vi "Periodic Tasks.vi"(8 "error in (no error)":errorcluster) -> ()   [LabVIEW 2023]
doc: "This VI runs in parallel to other tasks. It can contain as many user-defined periodic loops as you need. These can carry out PID or other sorts of timed response."
uses:
  Drive/DriveGlobal.vi
  <vilib>/Rock Robotics/Network Tables/NT Read String.vi
  <vilib>/Rock Robotics/Network Tables/NT Write Number.vi
  <vilib>/Rock Robotics/Network Tables/NT Write String.vi
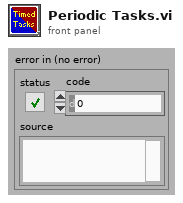
[diagram p1: front panel]
types:
  T1 = typedef "ADIS16470 Device Reference.ctl" = cluster{"DevStatus":errorcluster, "Hardware Config":T2, "Calibration Complete":refnum<notifier>, "Status Reference":refnum<data-value>, "Data Reference":refnum<data-value>, "Sychronous Process VI":T6, "Cmd FIFO":refnum<k33>, "Source":T7, "Data FIFO":refnum<k33>, "Calibration Time (ms)":u32, "Data Reference":refnum<data-value>}
  T2 = typedef "ADIS16470 Hardware Configuration.ctl" = cluster{"SPI Clock Rate (Hz)":dbl, "IMU SPI Mode (3)":T3, "IMU Reset Pin":T4, "IMU SPI Bus":T5, "IMU Data Ready Pin":T4, "Stall Config":cluster{"Pow2BytesPerRead":u8, "StallTicks":u16, "CsToSclkTicks":u8}}
  T3 = typedef "WPI_SPIMode.ctl" = enum16{"Mode 0 (Clk Idle Low,Sample on Leading)", "Mode 1 (Clk Idle Low,Sample on Trailing)", "Mode 2 (Clk Idle High,Sample on Leading)", "Mode 3 (Clk Idle High,Sample on Trailing)"}
  T4 = typedef "FPGA_DIOChannel.ctl" = enum8{"DIO 0", "DIO 1", "DIO 2", "DIO 3", "DIO 4", "DIO 5", "DIO 6", "DIO 7", "DIO 8", "DIO 9", "DIO MXP 0", "DIO MXP 1", "DIO MXP 2", "DIO MXP 3", "DIO MXP 4", "DIO MXP 5", "DIO MXP 6", "DIO MXP 7", "DIO MXP 8", "DIO MXP 9", "DIO MXP 10", "DIO MXP 11", "DIO MXP 12", "DIO MXP 13", "DIO MXP 14", "DIO MXP 15", "SPI Port CS1", "SPI Port CS2", "SPI Port CS3", "SPI Port MISO", "SPI Port MOSI", "Invalid"}
  T5 = typedef "spi_bus.ctl" = enum16{"SPI On-Board, CS0", "SPI On-Board, CS1", "SPI On-Board, CS2", "SPI On-Board, CS3", "SPI MXP", "Invalid"}
  T6 = typedef "ADIS16470 Process.ctl" = refnum<vi>
  T7 = typedef "FPGA_CounterEncoderSourceConvertionLVSourceType.ctl" = cluster{"DevStatus":errorcluster, "AnalogTriggerMode?":bool, "DigitalMode":cluster{"DIO Channel":T8}, "AnalogTriggerMode":cluster{"AnalogTriggerIndex":T9, "OutputType":T10}}
  T8 = typedef "FPGA_DIODigitalSourceChannel.ctl" = enum8{"DIO 0", "DIO 1", "DIO 2", "DIO 3", "DIO 4", "DIO 5", "DIO 6", "DIO 7", "DIO 8", "DIO 9", "DIO MXP 0", "DIO MXP 1", "DIO MXP 2", "DIO MXP 3", "DIO MXP 4", "DIO MXP 5", "DIO MXP 6", "DIO MXP 7", "DIO MXP 8", "DIO MXP 9", "DIO MXP 10", "DIO MXP 11", "DIO MXP 12", "DIO MXP 13", "DIO MXP 14", "DIO MXP 15", "SPI Port CS1", "SPI Port CS2", "SPI Port CS3", "SPI Port MISO", "SPI Port MOSI", "Disabled"}
  T9 = typedef "FPGA_AnalogTriggerIndex.ctl" = enum8{"Trig 0", "Trig 1", "Trig 2", "Trig 3", "Trig 4", "Trig 5", "Trig 6", "Trig 7", "Invalid"}
  T10 = typedef "FPGA_AnalogTriggerOutType.ctl" = enum16{"InWindow", "TriggerState", "Rising", "Falling"}
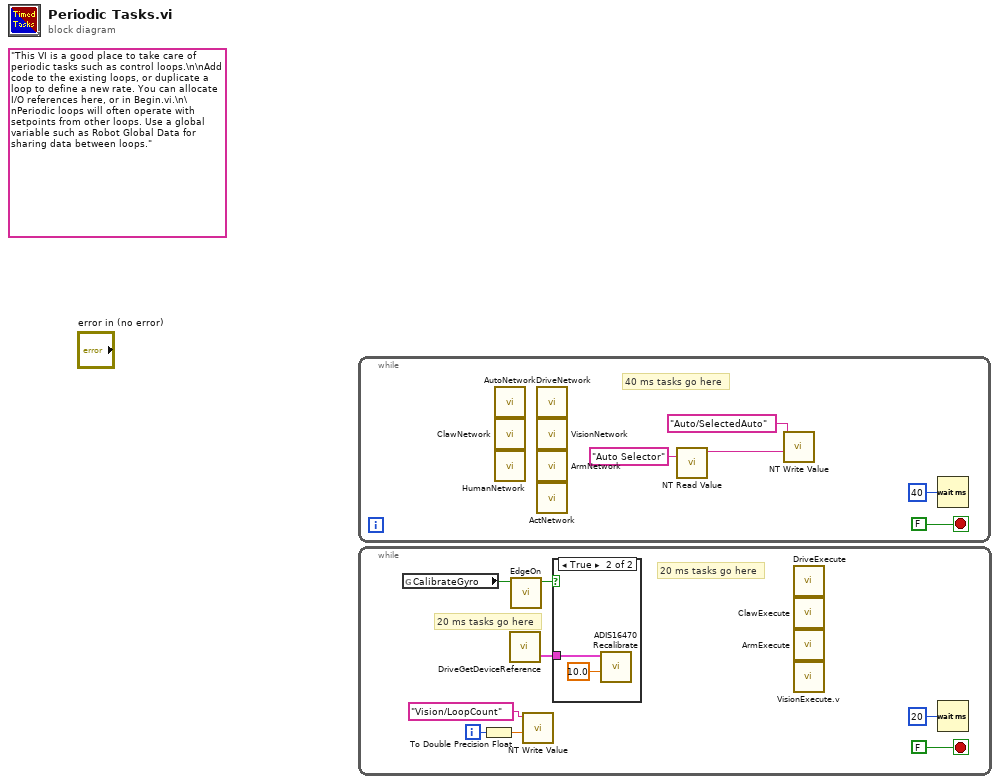
[diagram p0: block diagram]
diagram:
  (unwired) "This VI is a good place to take care of periodic tasks such as control loops.\n\nAdd code to the existing loops, or duplicate a loop to define a new rate. You can allocate I/O references here, or in Begin.vi.\n\nPeriodic loops will often operate with setpoints from other loops. Use a global variable such as Robot Global Data for sharing data between loops."
  n1 = while {
    stop <- FALSE stop-if-true
    # "40 ms tasks go here"
    n2 = call "AutoNetwork.vi"() -> ()  [unwired: 11 in, 1 out]
    n3 = call "ClawNetwork.vi"() -> ()  [unwired: 11 in, 1 out]
    n4 = call "HumanNetwork.vi"() -> ()  [unwired: 11 in, 1 out]
    n5 = call "DriveNetwork.vi"() -> ()  [unwired: 11 in, 1 out]
    n6 = call "VisionNetwork.vi"() -> ()  [unwired: 11 in, 1 out]
    n7 = call "ArmNetwork.vi"() -> ()  [unwired: 11 in, 1 out]
    n8 = call "ActNetwork.vi"() -> ()  [unwired: 11 in, 1 out]
    n9 = call-poly <vilib>:"NT Read Value.vi"("name"="Auto Selector" ("Name")) -> ("value"=w2:string)  [unwired: 8 in, 2 out]
    n10 = call-poly <vilib>:"NT Write Value.vi"("value"=w2, "name"="Auto/SelectedAuto") -> ()  [unwired: 9 in, 1 out]
    n11 = Wait (ms)(milliseconds to wait=u32 40) -> ()  [unwired: 1 out]
  }
  n12 = while {
    i -> [w6]
    stop <- FALSE stop-if-true
    # "20 ms tasks go here"
    # "20 ms tasks go here"
    n13 = global read "DriveGlobal.vi" "CalibrateGyro"() -> (w11:bool)
    n14 = To Double Precision Float(number=w6) -> (double precision float=w8:dbl)
    n15 = call "DriveGetDeviceReference.vi"() -> ("Gryo"=w10:T1)  [unwired: 11 in]
    n16 = call "EdgeOn.vi"("Current State"=w11) -> ("Edge On Found"=w9:bool)  [unwired: 10 in]
    n17 = call-poly <vilib>:"NT Write Value.vi"("value"=w8, "name"="Vision/LoopCount") -> ()  [unwired: 9 in, 1 out]
    n18 = case shown="True" w9 {
      tunnel: w10 -> [_ w14]
      frame False {
      }
      frame True {
        n19 = call <vilib>:"ADIS16470 Recalibrate.vi"("Calibration Time (4s)"=10.0, "ADIS16470DevRef in"=w14) -> ()  [unwired: 8 in, 2 out]
      }
    }
    n20 = call "DriveExecute.vi"() -> ()  [unwired: 11 in, 1 out]
    n21 = call "ClawExecute.vi"() -> ()  [unwired: 12 in]
    n22 = call "ArmExecute.vi"() -> ()  [unwired: 12 in]
    n23 = call "VisionExecute.v.vi"() -> ()  [unwired: 12 in]
    n24 = Wait (ms)(milliseconds to wait=u32 20) -> ()  [unwired: 1 out]
  }
